vi "event_register.vi"(8 "error in (no error)":errorcluster) -> (0 "error out":errorcluster, 3 "recipe":refnum<event-registration>)   [LabVIEW 2015, in "lv-recipe-machine.lvlib"]
uses:
  lv-recipe-machine.lvlib
  _controls/status.ctl
  _controls/mode.ctl
  _controls/manual_state.ctl
  _controls/automatic_state.ctl
  _controls/change.ctl
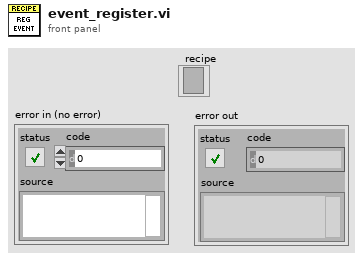
[diagram p1: front panel]
types:
  T1 = cluster{"status_event":refnum<user-event>, "change_out_event":refnum<user-event>}
  T2 = cluster{"status_event":bool, "change_out_event":bool}
  T3 = typedef "lv-recipe-machine.lvlib/references.ctl" = cluster{"semaphore":T4, "input_queue":refnum<queue>, "output_queue":refnum<queue>, "transition_queue":refnum<queue>, "data_dvr":refnum<data-value>, "stop_notifier":refnum<notifier>, "change_in_event":refnum<user-event>, "change_out_event":refnum<user-event>, "status_event":refnum<user-event>}
  T4 = typedef "Semaphore RefNum" = refnum<k1>
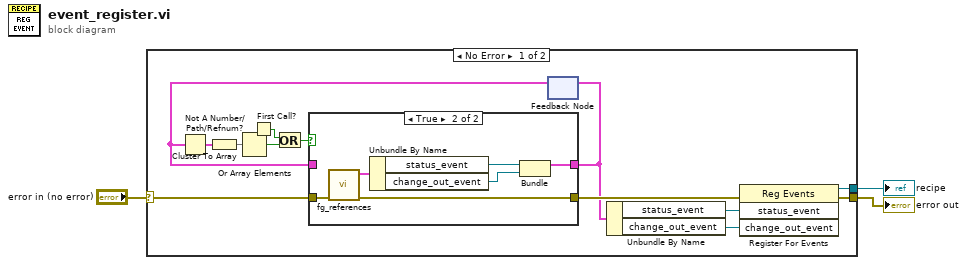
[diagram p0: block diagram]
diagram:
  n1 = case shown="No Error" "error in (no error)" {
    selector: "error in (no error)" -> [w12 w25]
    tunnel: [w10 w25] -> w2
    tunnel: [w4 _] -> w1
    frame No Error {
      n2 = First Call?() -> (First Call?: T/F=w14:bool)
      n3 = feedback #1() -> (w8:T1)  [unwired: 1 in]
      n4 = Not A Number/Path/Refnum?(number/path/refnum=w8) -> (NaN/Path/Refnum?=w15:T2)
      n5 = Cluster To Array(cluster=w15) -> (array=w7:bool[])
      n6 = Or Array Elements(Boolean array=w7) -> (logical OR=w9:bool)
      n7 = Or(x=w14, y=w9) -> (x .or. y?=w13:bool)
      n8 = case shown="True" w13 {
        tunnel: w12 -> [w17 w24]
        tunnel: [w17 w23] -> w16
        tunnel: [w18 w20] -> w11
        tunnel: w8 -> [w18 _]
        frame False {
        }
        frame True {
          n9 = call "fg_references.vi"("error in (no error)"=w24) -> ("error out"=w23:errorcluster, "references out"=w22:T3)  [unwired: 9 in]
          n10 = Unbundle By Name(w22) -> ("status_event"=w21:refnum<user-event>, "change_out_event"=w19:refnum<user-event>)
          n11 = Bundle("status_event"=w21, "change_out_event"=w19) -> (w20:T1)  [unwired: 1 in]
        }
      }
      n12 = feedback-in #1(w11) -> ()
      n13 = Unbundle By Name(w11) -> ("status_event"=w6:refnum<user-event>, "change_out_event"=w5:refnum<user-event>)
      n14 = register-events(error in=w16, w6, w5) -> (reference out=w4:refnum<event-registration>, error out=w10:errorcluster)  [unwired: 1 in]
    }
    frame Error {
    }
  }
  "error out" <- w2
  "recipe" <- w1
